vi "FPGA.vi"() -> ()   [LabVIEW 2014]
uses:
  <vilib>/rvi/Emulation/niFpgaGetClockAttributes.vi
  <vilib>/rvi/Emulation/niFpgaSctlEmulationGetInTimedLoop.vi
  <vilib>/rvi/Emulation/niFpgaEmulationReportErrorSimple.vi
  <vilib>/rvi/eio/common/nirviEmuTemplateMethod_errors.vi
  <vilib>/rvi/Emulation/niFpgaCriticalErrorInLSC.vi
  <vilib>/eio/EIONode/EIONode.xnode
panel:
  in  "Mod2/AO3":fxp<+/-,20,5>
  in  "Mod2/AO2":fxp<+/-,20,5>
  in  "Mod2/AO1":fxp<+/-,20,5>
  in  "Mod2/AO0":fxp<+/-,20,5>
  out "Mod1/AI3":fxp<+/-,24,4>
  out "Mod1/AI2":fxp<+/-,24,4>
  out "Mod1/AI1":fxp<+/-,24,4>
  out "Mod1/AI0":fxp<+/-,24,4>
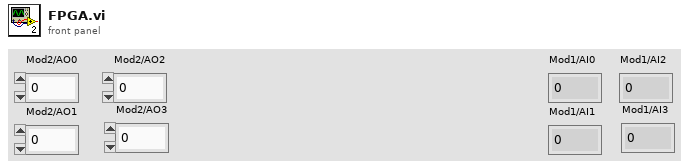
[diagram p1: front panel]
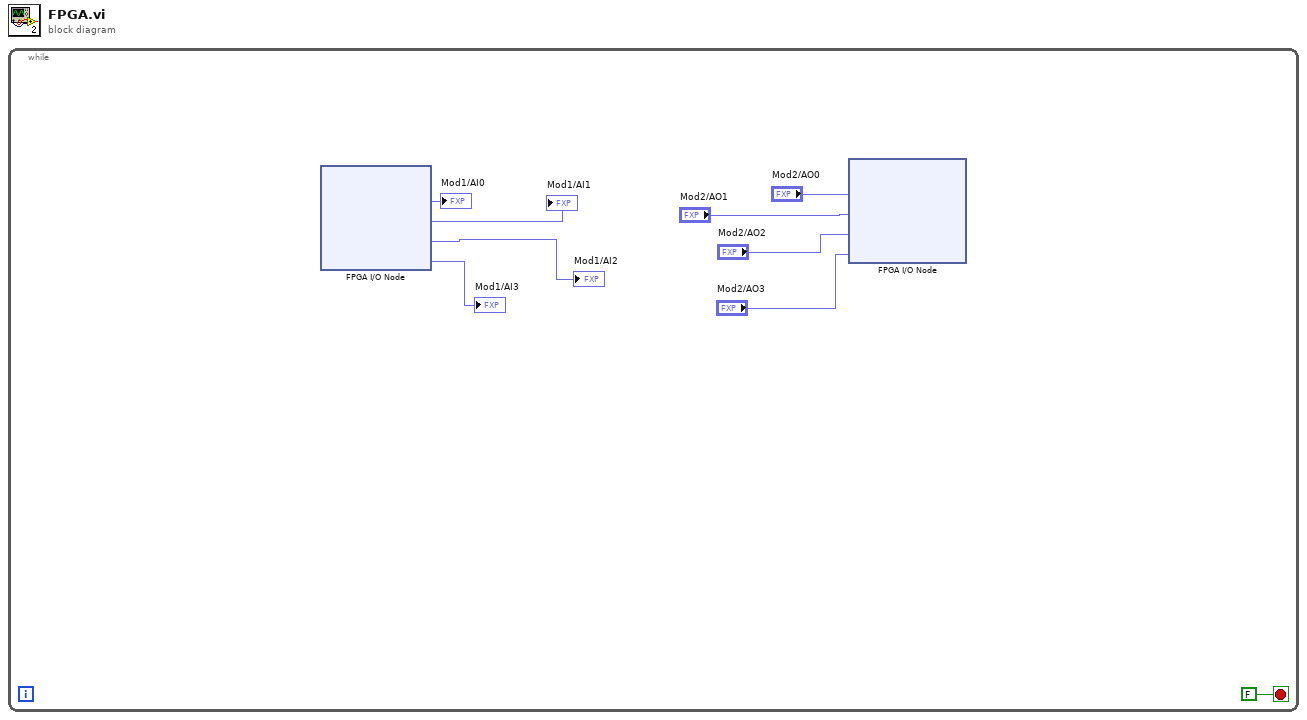
[diagram p0: block diagram]
diagram:
  n1 = while {
    stop <- FALSE stop-if-true
    n2 = xnode "FPGA I/O Node"() -> ("Mod1/AI0"=→"Mod1/AI0":fxp<+/-,24,4>, "Mod1/AI1"=→"Mod1/AI1":fxp<+/-,24,4>, "Mod1/AI2"=→"Mod1/AI2":fxp<+/-,24,4>, "Mod1/AI3"=→"Mod1/AI3":fxp<+/-,24,4>)  [unwired: 4 in, 4 out]
    n3 = xnode "FPGA I/O Node"("Mod2/AO0"="Mod2/AO0", "Mod2/AO1"="Mod2/AO1", "Mod2/AO2"="Mod2/AO2", "Mod2/AO3"="Mod2/AO3") -> ()  [unwired: 4 in, 4 out]
  }
